vi "Write Y.vi"(8 "error in (no error)":errorcluster, 10 "Y":dbl[](array[numeric]), 11 "Lockin Digitizer Driver in":refnum<class "Lockin Digitizer Driver.lvclass">) -> (0 "error out":errorcluster, 3 "Lockin Digitizer Driver out":refnum<class "Lockin Digitizer Driver.lvclass">)   [LabVIEW 2021, in "Lockin Digitizer Driver.lvclass"]
uses:
  Lockin Digitizer Driver.lvclass
  Lockin Digitizer Driver.lvclass/Lockin Digitizer Driver.ctl
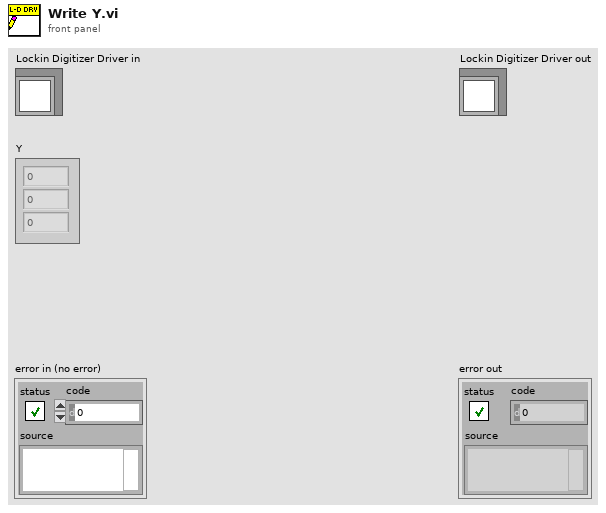
[diagram p1: front panel]
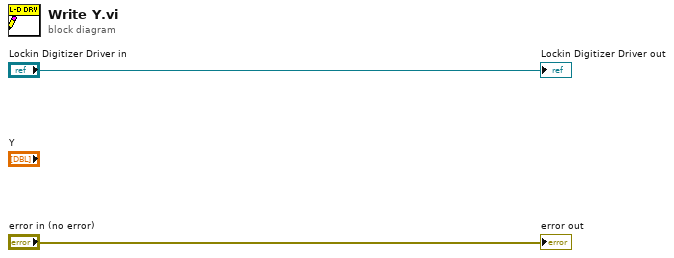
[diagram p0: block diagram]
diagram:
  "error out" <- "error in (no error)"
  "Lockin Digitizer Driver out" <- "Lockin Digitizer Driver in"
